vi "MKS_bla.vi"() -> ()   [LabVIEW 2009]
uses:
  <vilib>/Instr/_visa.llb/VISA Configure Serial Port (Instr).vi
panel:
  out "read buffer":string
  in  "write buffer":string
  in  "ms Wartezeit 2":u32=100
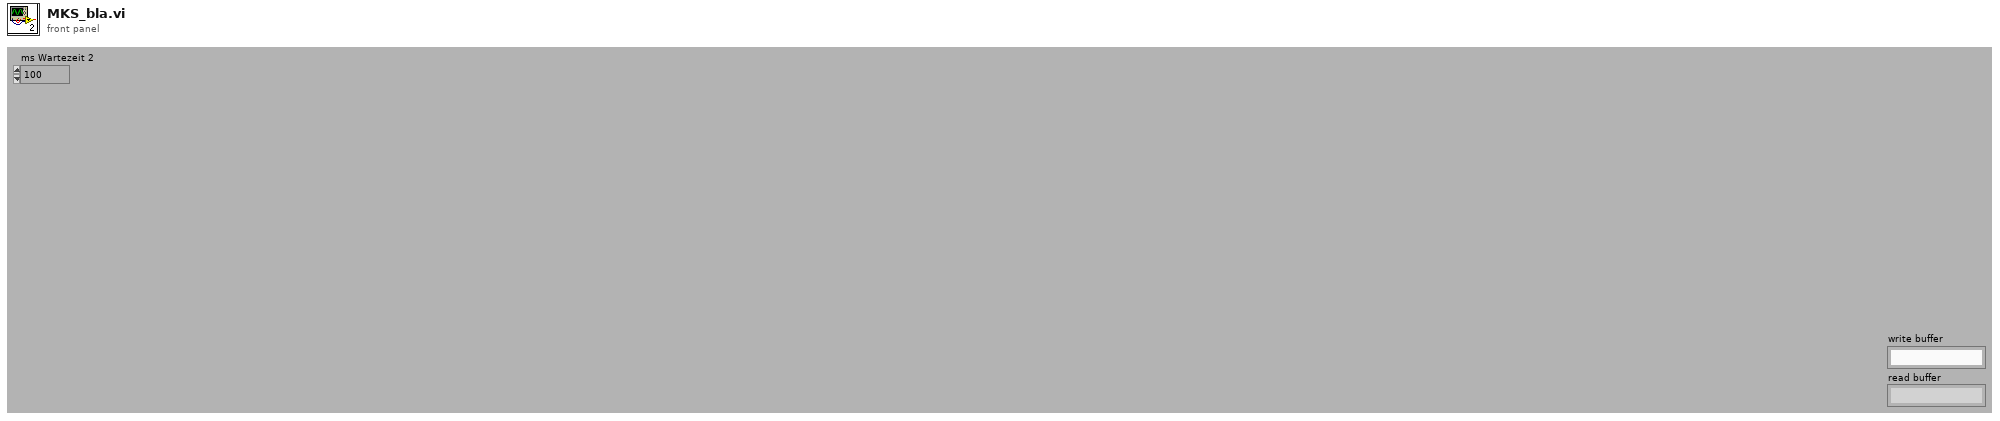
[diagram p1: front panel]
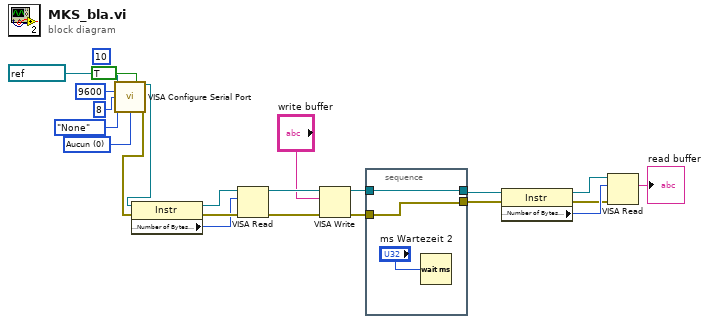
[diagram p0: block diagram]
diagram:
  w20 = u16 0 items=["Aucun", "XON/XOFF", "RTS/CTS", "XON/XOFF & RTS/CTS", "DTR/DSR", "XON/XOFF & DTR/DSR"] ("flow control (0:none)")
  (unwired) u8 10 ("termination char\n(0xA = '\\n' = LF)")
  n1 = call-poly "VISA Configure Serial Port"("VISA resource name"=refnum<visa-resource-name> "COM1", "Enable Termination\nChar (T)"=TRUE ("Enable Termination\nChar (T)"), "baud rate (9600)"=u32 9600, "data bits (8)"=u16 8, "parity (0:none)"=enum16{"None", "Odd", "Even", "Mark", "Space"}."None", "flow control (0:none)"=w20) -> ("VISA resource name out"=w21:refnum<visa-resource-name>, "error out"=w22:errorcluster)  [unwired: 8 in]
  n2 = property class="Instr"(reference=w21, error in=w22) -> (reference out=w4:refnum<visa-resource-name>, error out=w5:errorcluster, "Serial Settings:Number of Bytes at Serial Port"=w3:u32)
  n3 = VISA Read(VISA resource name=w4, byte count=w3, error in (no error)=w5) -> (VISA resource name out=w8:refnum<visa-resource-name>, error out=w9:errorcluster)  [unwired: 2 out]
  n4 = VISA Write(VISA resource name=w8, write buffer="write buffer", error in (no error)=w9) -> (VISA resource name out=w7:refnum<visa-resource-name>, error out=w6:errorcluster)  [unwired: 1 out]
  n5 = stacked-sequence {
    tunnel: [w25] -> w14
    tunnel: w6 -> [w25]
    tunnel: [w24] -> w13
    tunnel: w7 -> [w24]
    frame #0 {
      n6 = Wait (ms)(milliseconds to wait="ms Wartezeit 2") -> ()  [unwired: 1 out]
    }
  }
  n7 = property class="Instr"(reference=w13, error in=w14) -> (reference out=w11:refnum<visa-resource-name>, error out=w10:errorcluster, "Serial Settings:Number of Bytes at Serial Port"=w12:u32)
  n8 = VISA Read(VISA resource name=w11, byte count=w12, error in (no error)=w10) -> (read buffer=→"read buffer":string)  [unwired: 3 out]
